vi "识别手势.vi"(11 "Reconze  hands":T1) -> (0 "Item data":string[][](table)=[["1", "2017/2/3 22:44:49", "你好", "45", "0", "0", "0", "0", "0", "0", "0", "100"], ["2", "2017/2/3 22:57:09", "加油", "0", "90", "0", "0", "0", "0", "0", "0", "100"]], 1 "最小值":dbl, 2 "语义":string, 3 "ID":i32)   [LabVIEW 2016]
uses:
  Controls/recognize hands data.ctl
  Data Base/StateMachineStates.ctl
panel:
  out "元素索引":i32
  out "数组":dbl[](array[numeric])
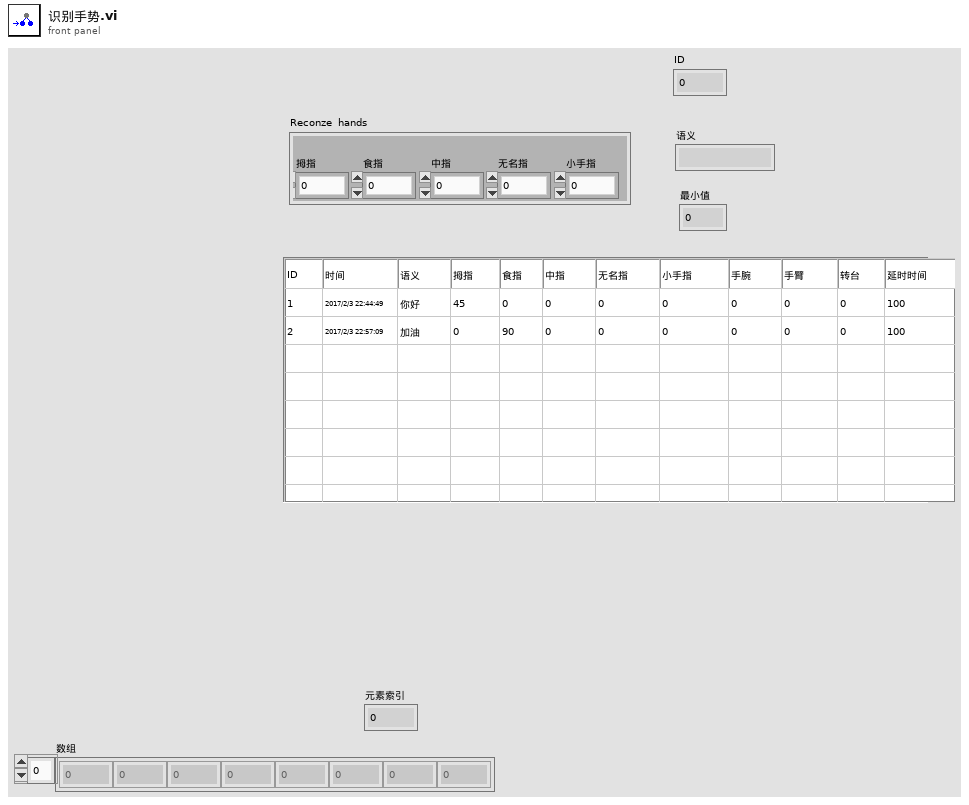
[diagram p1: front panel]
types:
  T1 = typedef "recognize hands data.ctl" = cluster{"小手指":sgl, "无名指":sgl, "中指":sgl, "食指":sgl, "拇指":sgl}
  T2 = cluster{"Time_Table":string, "Meaning":string, "Thumb":string, "arm":string, "delay":string, "Identity":string, "passport":string, "Index":string, "Middle":string, "ring":string, "little":string, "wrist":string, "rota":string, "Filename":string, "Table":string}
  T3 = typedef "StateMachineStates.ctl" = enum16{"Connection DB", "Creat DB", "Delete Table", "Insert DB", "Inquire Table", "Inquire All DB", "Delete All Data", "Delete Data", "Sort Data", "Inquire Last Data", ""}
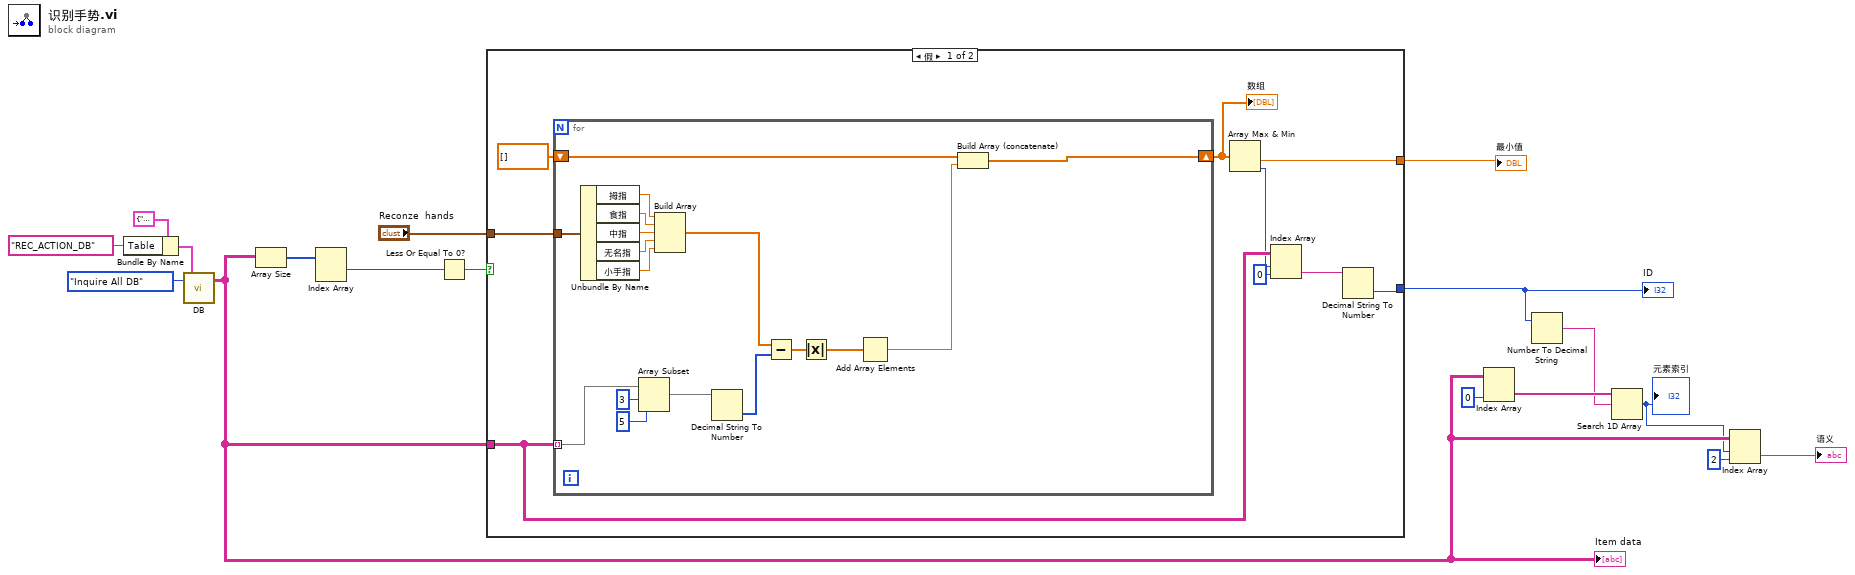
[diagram p0: block diagram]
diagram:
  n1 = Bundle By Name(cluster=T2 {"Time_Table"="时间", "Meaning"="语义", "Thumb"="拇指", "arm"="手臂", "delay"="延时时间", "Identity"="ID", "passport"="", "Index"="食指", "Middle"="中指", "ring"="无名指", "little"="小手指", "wrist"="手腕", "rota"="转台", "Filename"="PZJData.mdb", "Table"="ACTION_DB"} ("Data Table"), "Table"="REC_ACTION_DB") -> (w15:T2)
  n2 = call "DB.vi"("Beginning State"=StateMachineStates."Inquire All DB", "Data Table"=w15) -> ("Item Data"=w8:string[][])  [unwired: 11 in, 6 out]
  "Item data" <- w8
  n3 = Array Size(array=w8) -> (size(s)=w12:i32[])
  n4 = Index Array(array=w12) -> (element #1=w13:i32)  [unwired: 2 in, 1 out]
  n5 = Less Or Equal To 0?(x=w13) -> (x <= 0?=w11:bool)
  n6 = case shown="假" w11 {
    tunnel: w8 -> [w22 _]
    tunnel: "Reconze  hands" -> [w26 _]
    tunnel: [w20 _] -> w10
    tunnel: [w18 _] -> w5
    frame False {
      n7 = for {
        tunnel: w22 -> [w40] mode=indexing
        tunnel: w26 -> [w43]
        shift-right: [w27] -> w24
        shift-left: dbl[] [] -> [w29]
        n8 = Unbundle By Name(w43) -> ("拇指"=w38:sgl, "食指"=w37:sgl, "中指"=w36:sgl, "无名指"=w35:sgl, "小手指"=w34:sgl)
        n9 = Array Subset(array=w40, index=3 ("索引"), length=5 ("长度")) -> (w39:string[])
        n10 = Build Array(w38, w37, w36, w35, w34) -> (w33:sgl[])
        n11 = Decimal String To Number(string=w39) -> (number=w32:i32[])  [unwired: 2 in, 1 out]
        n12 = Subtract(x=w33, y=w32) -> (x-y=w31:sgl[])
        n13 = Absolute Value(x=w31) -> (abs(x)=w30:sgl[])
        n14 = Add Array Elements(numeric array=w30) -> (sum=w28:sgl)
        n15 = Build Array (concatenate)(w29, w28) -> (w27:dbl[])
      }
      "数组" <- w24
      n16 = Array Max & Min(array=w24) -> (min value=w20:dbl, min index (indices)=w21:i32)  [unwired: 2 out]
      n17 = Index Array(array=w22, index (row)=w21, index (col)=0 ("禁用的索引 (列)")) -> (element=w19:string)
      n18 = Decimal String To Number(string=w19) -> (number=w18:i32)  [unwired: 2 in, 1 out]
    }
    frame True {
    }
  }
  "最小值" <- w10
  "ID" <- w5
  n19 = Index Array(array=w8, index (col)=0 ("禁用的索引 (列)")) -> (element=w6:string[])  [unwired: 1 in]
  n20 = Number To Decimal String(number=w5) -> (decimal integer string=w4:string)  [unwired: 1 in]
  n21 = Search 1D Array(1D array=w6, element=w4) -> (index of element=w3:i32)  [unwired: 1 in]
  "元素索引" <- w3
  n22 = Index Array(array=w8, index (row)=w3, index (col)=2 ("禁用的索引 (列)")) -> (element=→"语义":string)
